vi "Compute DistanceTo AprilTag using NI Apriltage Info.vi"(4 "Camera#":i32, 8 "Internal Parameters":T1, 11 "tag info":T2) -> (0 "Target Info":dbl[](array[numeric]), 2 "Tag Center Distance (in)":dbl, 3 "results out":T3={"diameter points"={"first point"={"x"=0.0, "y"=0.0}, "projected point"={"x"=0.0, "y"=0.0}}, "Tag Center"={"X"=0.0, "Y"=0.0}, "AprilTag #"=68, "homography matrix"=[], "corner points"=[]} {"Tag Center"."Y" format="%0.2f"; "Tag Center"."X" format="%0.2f"})   [LabVIEW 2025]
doc: "Using the camera lens information and the real world size of the target, use trig and ratios to determine the distance to the target. Also returns the location relative to the image center in a (-1 , 1) coordinate system that may be useful for steering the robot."
uses:
  AprilTag Target Fields.ctl
  <vilib>/vision/Calibration.llb/Internal Parameters.ctl
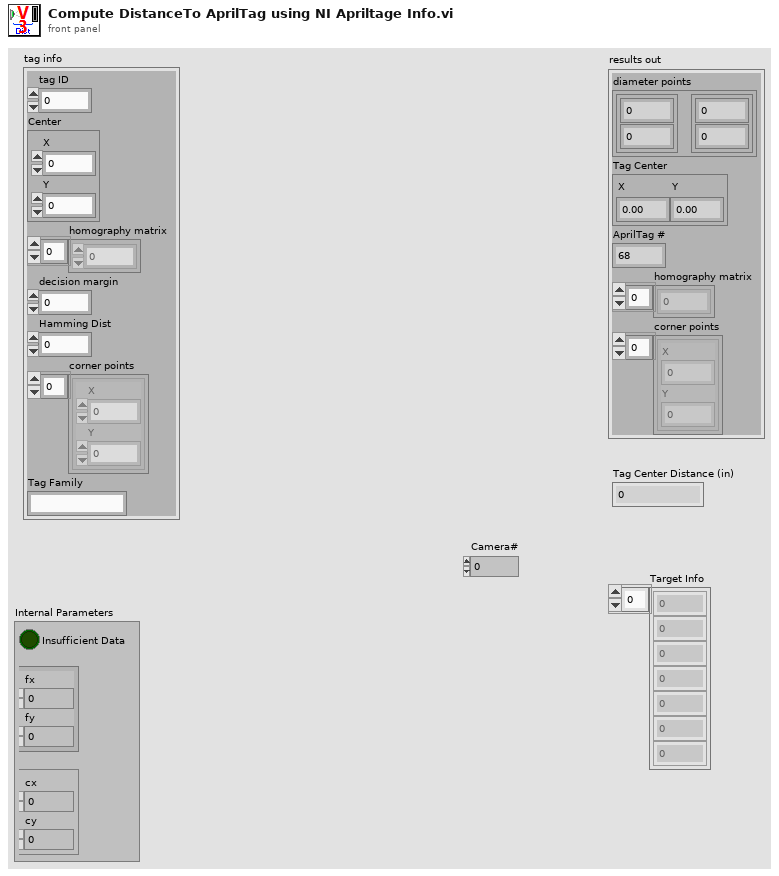
[diagram p1: front panel]
types:
  T1 = typedef "Internal Parameters.ctl" = cluster{"Insufficient Data":bool, "Focal Length (pixel)":cluster{"fx":sgl, "fy":sgl}, "Optical Center (pixel)":cluster{"cx":sgl, "cy":sgl}}
  T2 = cluster{"tag ID":i32, "Center":cluster{"X":dbl, "Y":dbl}, "homography matrix":dbl[], "decision margin":dbl, "Hamming Dist":i32, "corner points":cluster{"X":dbl, "Y":dbl}[], "Tag Family":string}
  T3 = typedef "AprilTag Target Fields.ctl" = cluster{"diameter points":cluster{"first point":cluster{"x":dbl, "y":dbl}, "projected point":cluster{"x":dbl, "y":dbl}}, "Tag Center":cluster{"X":dbl, "Y":dbl}, "AprilTag #":i32, "homography matrix":dbl[], "corner points":cluster{"X":dbl, "Y":dbl}[]}
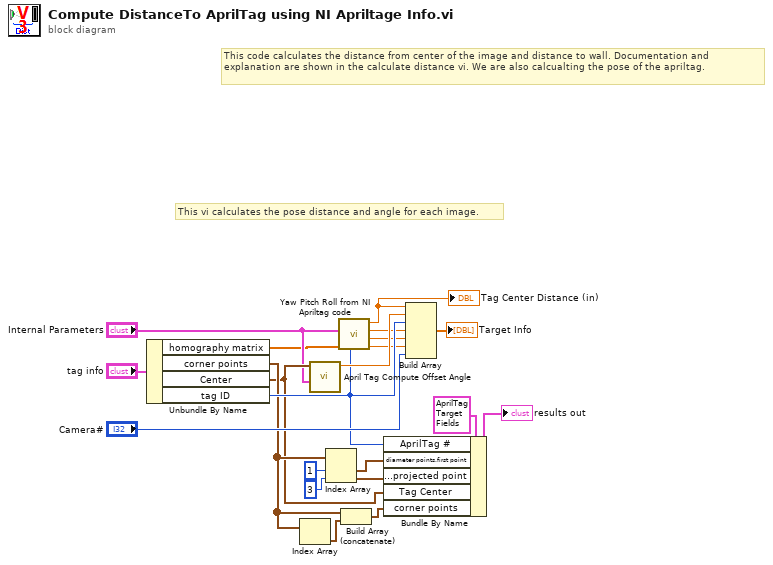
[diagram p0: block diagram]
diagram:
  # "This vi calculates the pose distance and angle for each image."
  # "This code calculates the distance from center of the image and distance to wall. Documentation and explanation are shown in the calculate distance vi. We are also calcualting the pose of the apriltag."
  n1 = Unbundle By Name("tag info") -> ("homography matrix"=w1:dbl[], "corner points"=w6:cluster{"X":dbl, "Y":dbl}[], "Center"=w3:cluster{"X":dbl, "Y":dbl}, "tag ID"=w11:i32)
  n2 = Index Array(array=w6) -> (element=w5:cluster{"X":dbl, "Y":dbl})  [unwired: 1 in]
  n3 = call "April Tag Compute Offset Angle.vi"("Internal Parameters"="Internal Parameters", "Tag Center"=w3) -> ("Bearing"=w14:dbl)  [unwired: 9 in]
  n4 = Index Array(array=w6, index #1=1 ("index"), index #2=3 ("index")) -> (element #1=w18:cluster{"X":dbl, "Y":dbl}, element #2=w17:cluster{"X":dbl, "Y":dbl})
  n5 = call "Yaw Pitch Roll from NI Apriltag code.vi"("Tag ID"=w11, "Homography H"=w1, "Internal Parameters"="Internal Parameters") -> ("Roll"=w8:dbl, "Pitch"=w9:dbl, "Yaw"=w10:dbl, "Tag Center Distance (in)"=w4:dbl)  [unwired: 5 in]
  "Tag Center Distance (in)" <- w4
  n6 = Build Array (concatenate)(w6, w5) -> (w7:cluster{"X":dbl, "Y":dbl}[])
  n7 = Bundle By Name(cluster=T3 {"diameter points"={"first point"={"x"=0.0, "y"=0.0}, "projected point"={"x"=0.0, "y"=0.0}}, "Tag Center"={"X"=408.5405926665837, "Y"=290.20374811802037}, "AprilTag #"=6, "homography matrix"=[80.20543116083331, -9.380219557443908, 408.5405926665837, 1.224067205918844, 70.26117200161627, 290.20374811802037, 0.00402105019898838, -0.03127119238049826, 1.0], "corner points"=[]} ("results out"), "AprilTag #"=w11, "diameter points.first point"=w18, "diameter points.projected point"=w17, "Tag Center"=w3, "corner points"=w7) -> (→"results out":T3)
  n8 = Build Array(w4, w14, w11, w10, w9, w8, "Camera#") -> (→"Target Info":dbl[])
